vi "Calculate Cycle Time.vi"(8 "error in (no error)":errorcluster, 11 "Coordinates":T1[](array[typedef]) {"Apparent Frame Size" format="%#_6f"; "Original FOV (um)" format="%#_6f"; "Pixels per miniscan" format="%#_6f"; "Dwell Time per pixel" format="%#_6f"; "Resolution" format="%#_6f"; "ROI group ID" format="%#_6f"; "Laser Power (%)" format="%#_6f"; "Zoom" format="%#_6f"; "Frame Size" format="%#_6f"; "Number of lines" format="%#_6f"; "Composite ID" format="%#_6f"; "Angle (deg)" format="%#_6f"; "ROI Time (ns)" format="%#_6f"; "ROI ID" format="%#_6f"; "Pixels in ROI" format="%#_6f"; "ROI index" format="%#_6f"; "Z stop" format="%#_6f"; "Y stop" format="%#_6f"; "X stop" format="%#_6f"; "Z start" format="%#_6f"; "X start" format="%#_6f"; "Y start" format="%#_6f"}) -> (0 "error out":errorcluster, 1 "AOD fill time (us)":dbl=24.16, 2 "Cycle time (us)":dbl)   [LabVIEW 2020]
uses:
  Visualisation/Functional Imaging Viewer/Typedefs/ROI parameters data type.ctl
  Typedefs/ROI ID Enum.ctl
  Global Variables/General Globals.vi
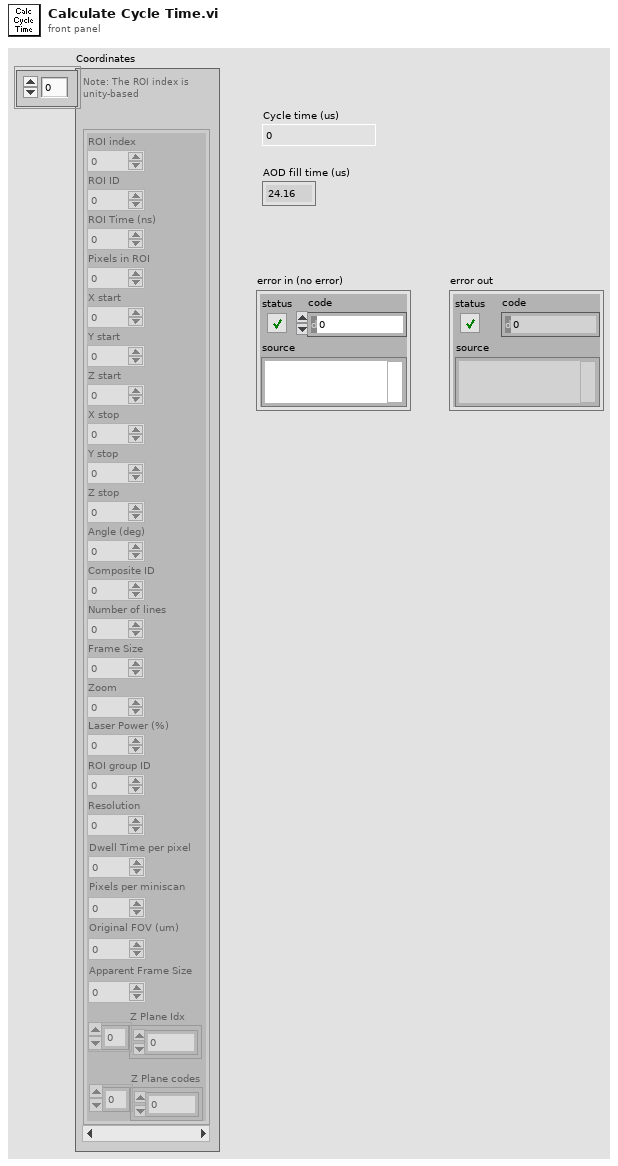
[diagram p1: front panel]
types:
  T1 = typedef "ROI parameters data type.ctl" = cluster{"ROI index":dbl, "ROI ID":dbl, "ROI Time (ns)":dbl, "Pixels in ROI":dbl, "X start":dbl, "Y start":dbl, "Z start":dbl, "X stop":dbl, "Y stop":dbl, "Z stop":dbl, "Angle (deg)":dbl, "Composite ID":dbl, "Number of lines":dbl, "Frame Size":dbl, "Zoom":dbl, "Laser Power (%)":dbl, "ROI group ID":dbl, "Resolution":dbl, "Dwell Time per pixel":dbl, "Pixels per miniscan":dbl, "Original FOV (um)":dbl, "Apparent Frame Size":dbl, "Z Plane Idx":i32[], "Z Plane codes":i32[]}
  T2 = typedef "ROI ID Enum.ctl" = enum16{"Point", "MiniScan", "Comp. MiniScan", "Rectangle", "Comp. volume", "Arb. plane point", "None"}
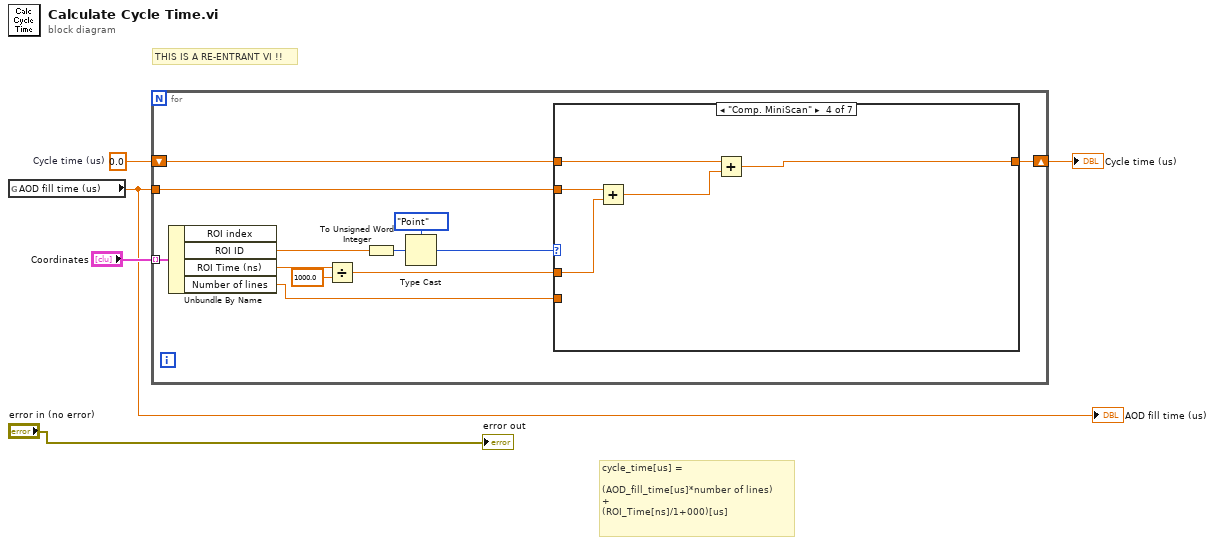
[diagram p0: block diagram]
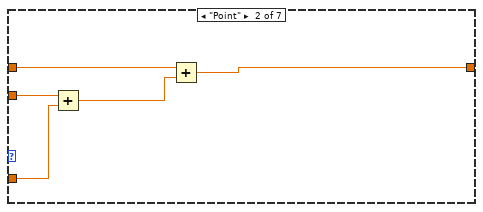
[diagram p3: hidden frame]
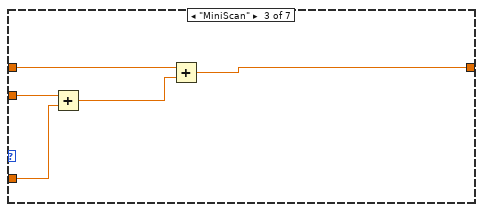
[diagram p4: hidden frame]
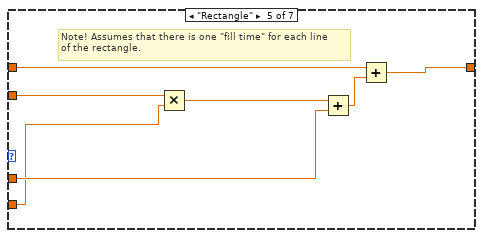
[diagram p5: hidden frame]
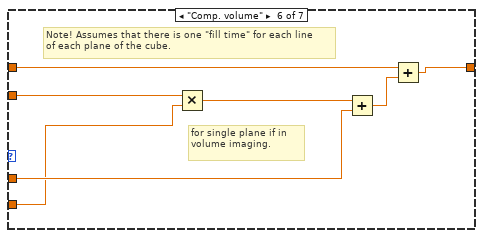
[diagram p6: hidden frame]
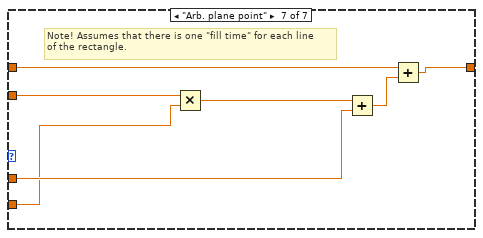
[diagram p7: hidden frame]
diagram:
  w4 = 0.0  # Cycle time (us)
  # "cycle_time[us] = \n\n(AOD_fill_time[us]*number of lines) \n+ \n(ROI_Time[ns]/1+000)[us]"
  # "THIS IS A RE-ENTRANT VI !!"
  n1 = global read "General Globals.vi" "AOD fill time (us)"() -> (w3:dbl)
  "AOD fill time (us)" <- w3
  n2 = for {
    tunnel: "Coordinates" -> [w17] mode=indexing
    tunnel: w3 -> [w16]
    shift-right: [w15] -> w2
    shift-left: w4 -> [w14]
    n3 = Unbundle By Name(w17) -> ("ROI ID"=w13:dbl, "ROI Time (ns)"=w8:dbl, "Number of lines"=w6:dbl)  [unwired: 1 out]
    n4 = Divide(x=w8, y=1000.0) -> (x/y=w7:dbl)
    n5 = To Unsigned Word Integer(number=w13) -> (unsigned 16bit integer=w11:u16)
    n6 = Type Cast(type=ROI_ID_Enum."Point" ("ROI ID Enum"), x=w11) -> (*(type *) &x=w10:T2)
    n7 = case shown="\"Rectangle\"" w10 {
      tunnel: w7 -> [_ w23 w28 w33 w40 w47 w54]
      tunnel: w16 -> [_ w22 w27 w32 w36 w43 w50]
      tunnel: [w18 w21 w26 w31 w39 w46 w53] -> w15
      tunnel: w14 -> [w18 w20 w25 w30 w38 w45 w52]
      tunnel: w6 -> [_ _ _ _ w34 w42 w48]
      frame Default {
      }
      frame "Point" {
        n8 = Add(x=w22, y=w23) -> (x+y=w19:dbl)
        n9 = Add(x=w20, y=w19) -> (x+y=w21:dbl)
      }
      frame "MiniScan" {
        n10 = Add(x=w27, y=w28) -> (x+y=w24:dbl)
        n11 = Add(x=w25, y=w24) -> (x+y=w26:dbl)
      }
      frame "Comp. MiniScan" {
        n12 = Add(x=w32, y=w33) -> (x+y=w29:dbl)
        n13 = Add(x=w30, y=w29) -> (x+y=w31:dbl)
      }
      frame "Rectangle" {
        # "Note! Assumes that there is one \"fill time\" for each line\nof the rectangle."
        n14 = Multiply(x=w36, y=w34) -> (x*y=w35:dbl)
        n15 = Add(x=w35, y=w40) -> (x+y=w37:dbl)
        n16 = Add(x=w38, y=w37) -> (x+y=w39:dbl)
      }
      frame "Comp. volume" {
        # "for single plane if in volume imaging."
        # "Note! Assumes that there is one \"fill time\" for each line\nof each plane of the cube."
        n17 = Multiply(x=w43, y=w42) -> (x*y=w41:dbl)
        n18 = Add(x=w41, y=w47) -> (x+y=w44:dbl)
        n19 = Add(x=w45, y=w44) -> (x+y=w46:dbl)
      }
      frame "Arb. plane point" {
        # "Note! Assumes that there is one \"fill time\" for each line\nof the rectangle."
        n20 = Multiply(x=w50, y=w48) -> (x*y=w49:dbl)
        n21 = Add(x=w49, y=w54) -> (x+y=w51:dbl)
        n22 = Add(x=w52, y=w51) -> (x+y=w53:dbl)
      }
    }
  }
  "Cycle time (us)" <- w2
  "error out" <- "error in (no error)"
